vi "MVMT.vi"() -> ()   [LabVIEW 2011]
uses:
  <vilib>/vision/Pattern Matching.llb/IMAQ Curve Parameters.ctl
  <vilib>/vision/Analysis.llb/IMAQ ExtractCurvesCurve.ctl
  <vilib>/Platform/TimedLoop/XDataNode/timing_clust.ctl
  <vilib>/Platform/TimedLoop/XDataNode/nitl_modes.ctl
  <vilib>/Platform/TimedLoop/XDataNode/wakeup.ctl
  <vilib>/Platform/TimedLoop/XDataNode/XDataNode.xnode
  <vilib>/vision/NI_Vision_Development_Module.lvlib
  <vilib>/Platform/TimedLoop/XDataNode/XDNodeRunTimeDep.lvlib
panel:
  in  "Median Filter Size":i32=5 min=0 max=7
  in  "Distance to Camera Visible":cluster{dbl, dbl}(slide)={0.0, 3.88} scale=0.0..3.0
  out "Curves":T1[](array[typedef]) {"Points"."Y" format="%.2f"; "Points"."X" format="%.2f"}
  out "Image":T2(plugin-control)
  in  "Curve Parameters":T3={"Extraction Mode"=1, "Edge Threshold"=1, "Edge Filter Size"=0, "Min Length"=25, "Row Search Step Size"=15, "Col Search Step Size"=15, "Max Endpoint Gap"=10, "Closed"=TRUE, "Subpixel"=TRUE} {"Extraction Mode" items=["Normal", "Uniform Regions"]; "Edge Filter Size" items=["Fine", "Normal", "Contour Tracing"]; "Max Endpoint Gap" min=0; "Col Search Step Size" min=1 max=255 step=1; "Row Search Step Size" min=1 max=255 step=1; "Min Length" min=0; "Edge Threshold" min=1 max=350 step=1}
  in  "Range":cluster{"Lower value":sgl, "Upper value":sgl}={"Lower value"=0.05, "Upper value"=10.0} {"Upper value" format="%.2f"; "Lower value" format="%.2f"}
  in  "Zero Out Baseline":bool
  in  "Status":string
  in  "Start":bool
  out "Frame Display":T2(plugin-control)
  in  "# Frames in Average":i32=100
  in  "stop":bool
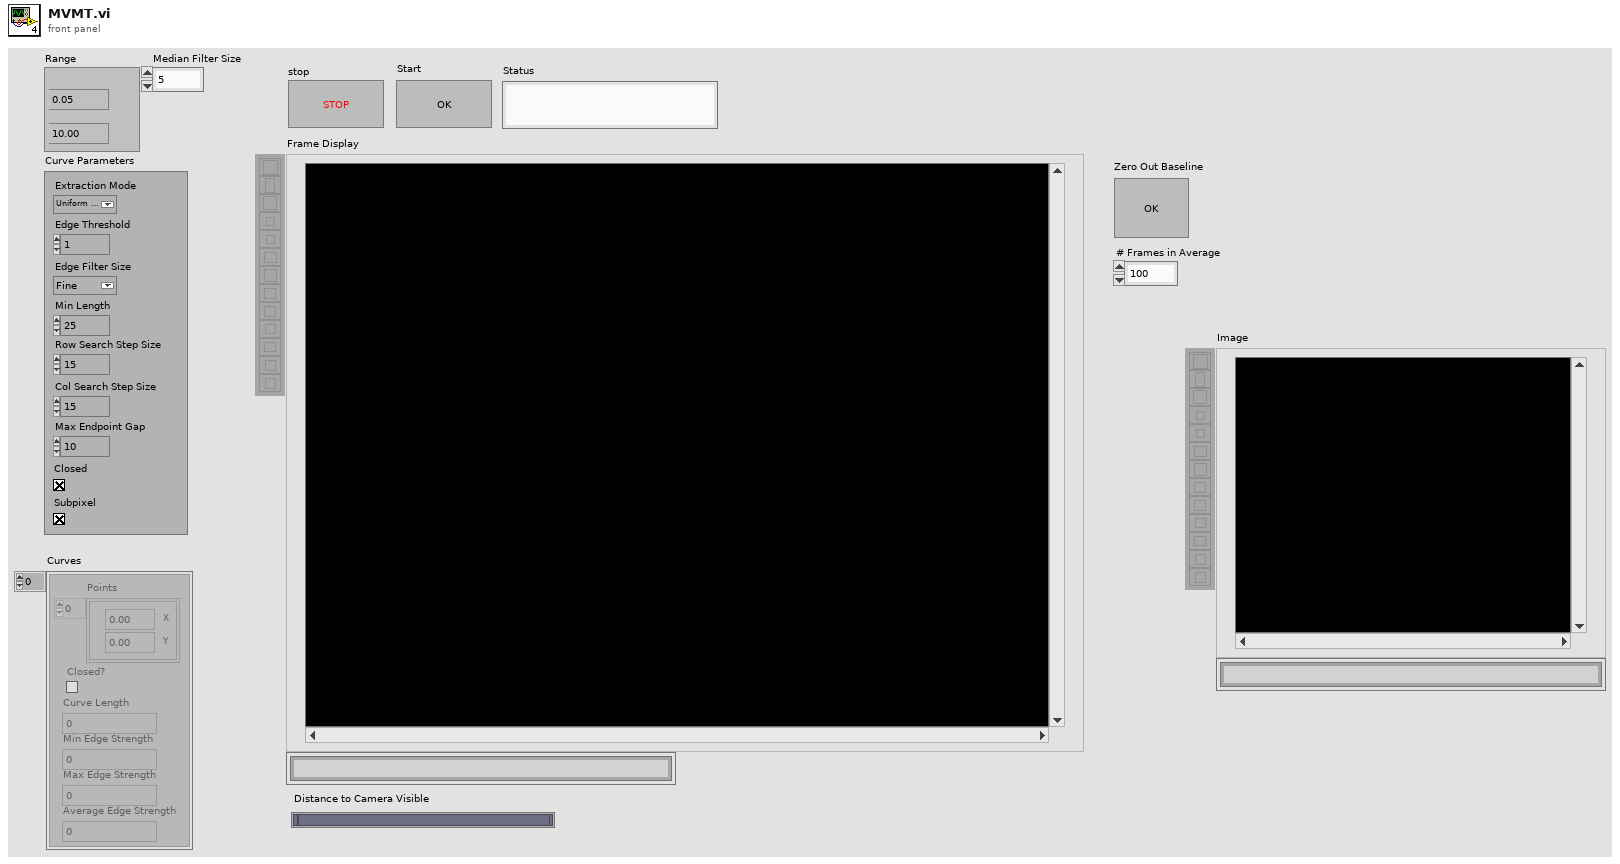
[diagram p1: front panel]
types:
  T1 = typedef "IMAQ ExtractCurvesCurve.ctl" = cluster{"Points":cluster{"X":dbl, "Y":dbl}[], "Closed?":bool, "Curve Length":dbl, "Min Edge Strength":dbl, "Max Edge Strength":dbl, "Average Edge Strength":dbl}
  T2 = typedef "IMAQ Image.ctl" = refnum<image>
  T3 = typedef "IMAQ Curve Parameters.ctl" = cluster{"Extraction Mode":u32, "Edge Threshold":i32, "Edge Filter Size":u32, "Min Length":i32, "Row Search Step Size":i32, "Col Search Step Size":i32, "Max Endpoint Gap":i32, "Closed":bool, "Subpixel":bool}
  T4 = enum16{"Record", "Idle", "Acquire Background", "Stop"}
  T5 = typedef "t_CallbackReferences.ctl" = cluster{"LV event callback ":refnum<k27>, "Proxy instance":refnum<k24>, "(*f)(...)":i32}
  T6 = typedef "XDNodeRunTimeDep.lvlib/timing_clust.ctl" = cluster{"Expected End [f-1]":u64, "Actual End [f-1]":u64, "Finished Late? [f-1]":bool, "Expected End [i-1]":u64, "Actual End [i-1]":u64, "Finished Late? [i-1]":bool, "Expected Start [i]":u64, "Actual Start [i]":u64, "Expected Start [f]":u64, "Actual Start [f]":u64, "Source Name":string, "Structure Name":string, "Period":i64, "Deadline":i64, "Offset":i64, "Start":i64, "Priority":i32, "Timeout":i32, "Mode":T7, "Wakeup Reason":T8, "Error":errorcluster, "Source Type":string, "Secondary Source Type":string, "Global End Time":u64, "Global Start Time":u64, "Frame Duration":u64, "Iteration Duration":u64, "Assigned CPU":i32, "I/O Scan Engine Mode":u32}
  T7 = typedef "XDNodeRunTimeDep.lvlib/nitl_modes.ctl" = enum32{"No Change", "Process missed periods, maintain original phase", "Discard missed periods, maintain original phase", "Process missed periods, ignore original phase", "Discard missed periods, ignore original phase"}
  T8 = typedef "XDNodeRunTimeDep.lvlib/wakeup.ctl" = enum32{"Normal", "Aborted", "Asynchronous wakeup", "Timing source error", "Timed loop error", "Timeout"}
  T9 = enum32{"Average", "Min", "Max", "Clear  if < ", "Clear  if < or =", "Clear  if =", "Clear  if > or =", "Clear  if >"}
  T10 = typedef "Image Type" = u32
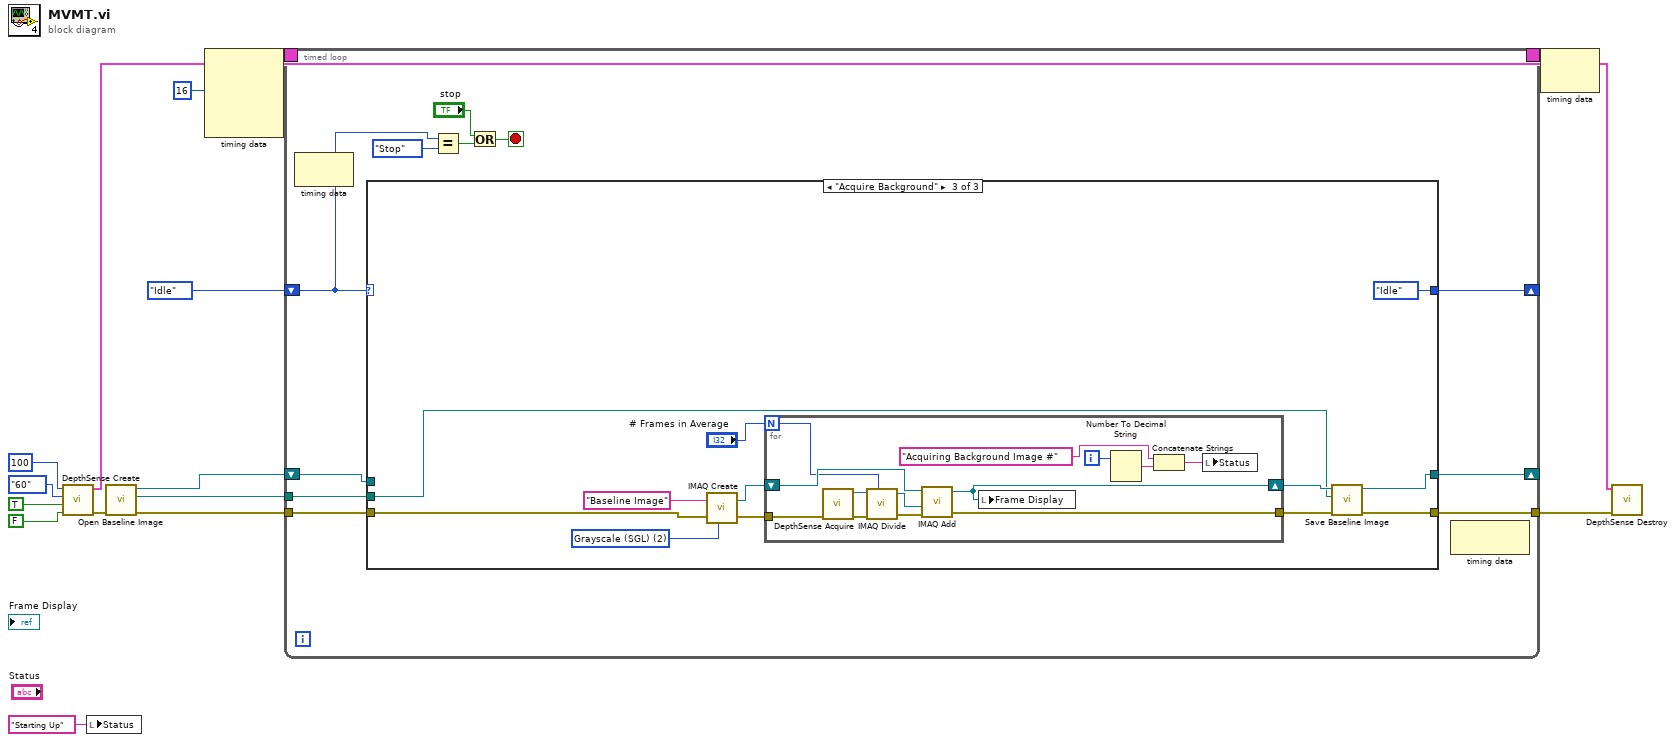
[diagram p0: block diagram]
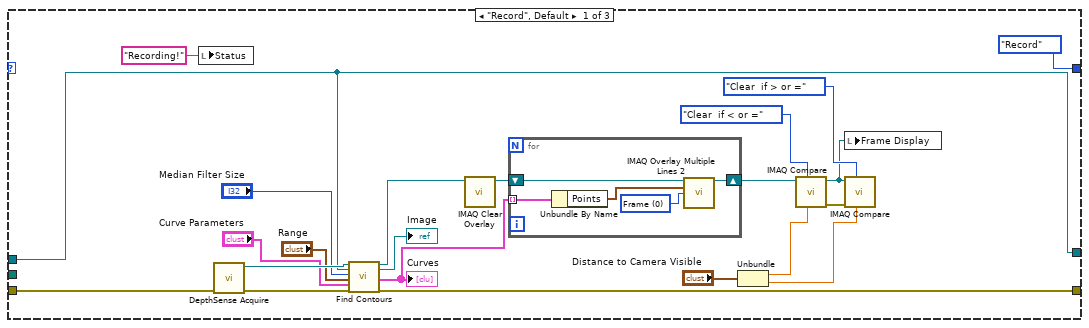
[diagram p2: hidden frame]
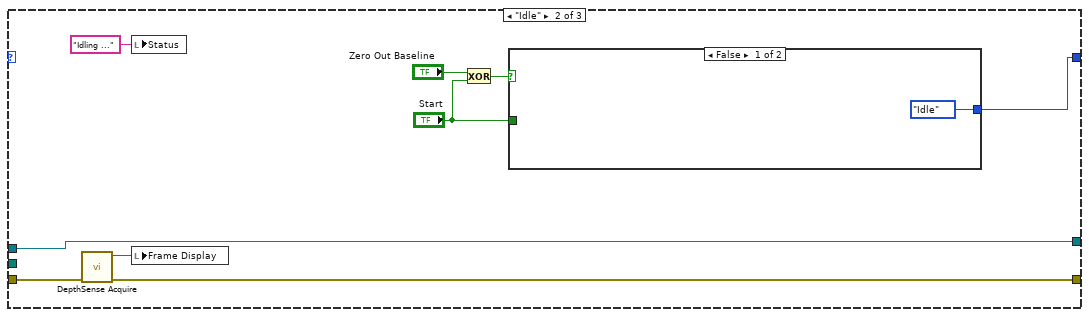
[diagram p3: hidden frame]
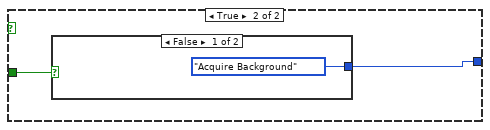
[diagram p4: hidden frame]
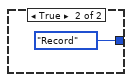
[diagram p5: hidden frame]
diagram:
  n1 = call "DepthSense Create.vi"("Denoise?"=FALSE, "Close Mode?"=TRUE, "Framerate"=enum32{"25", "30", "50", "60"}."60", "Confidence"=100) -> ("error out"=w5:errorcluster, "callbacks"=w1:cluster{"References":T5, "References":T5})  [unwired: 5 in, 1 out]
  n2 = local write "Status"("Starting Up" ("Status")) -> ()
  n3 = call "Open Baseline Image.vi"("error in (no error)"=w5) -> ("error out"=w4:errorcluster, "dup path"=w3:path, "Image Out"=w2:T2)  [unwired: 8 in]
  n4 = node-c288(i64 16 ("Period")) -> (w9:T6)  [unwired: 3 in]
  n5 = timed-loop {
    tunnel: w4 -> [w26]
    tunnel: [w25] -> w15
    shift-right: [w18] -> _
    shift-left: T4."Idle" -> [w20]
    shift-right: [w17] -> _
    shift-left: w2 -> [w24]
    tunnel: w3 -> [w16]
    timing: w9 -> [_]
    timing-out: [_] -> w8
    stop <- w22 stop-if-true
    n6 = node-c288() -> ()  [unwired: 1 in, 1 out]
    n7 = case shown="\"Acquire Background\"" w20 {
      tunnel: w26 -> [w50 w64 w77]
      tunnel: [w48 w63 w73] -> w25
      tunnel: w24 -> [w43 w61 _]
      tunnel: [T4."Record" w57 T4."Idle"] -> w18
      tunnel: [w43 w61 w70] -> w17
      tunnel: w16 -> [_ _ w71]
      frame "Record", Default {
        n8 = local write "Status"("Recording!" ("Status")) -> ()
        n9 = call "DepthSense Acquire.vi"("error in (no error)"=w50) -> ("error out"=w44:errorcluster, "new depth frame"=w47:T2)  [unwired: 9 in]
        n10 = call "Find Contours.vi"("Image Src"=w47, "Background Image"=w43, "Median Filter Size"="Median Filter Size", "Range"="Range", "Curve Parameters"="Curve Parameters", "error in (no error)"=w44) -> ("Image Src Dup"=w42:T2, "Background Subtracted Image"=→"Image":T2, "Curves"=w39:T1[], "error out"=w48:errorcluster)  [unwired: 10 in]
        "Curves" <- w39
        n11 = call "IMAQ Clear Overlay"("Image"=w42) -> ("Image Out"=w41:T2)  [unwired: 9 in, 1 out]
        n12 = for {
          tunnel: w39 -> [w55] mode=indexing
          shift-right: [w51] -> w38
          shift-left: w41 -> [w54]
          w52 = u32 0 items=["Frame", "Fill"] ("Drawing Mode (Frame)")
          n13 = Unbundle By Name(w55) -> ("Points"=w53:cluster{"X":dbl, "Y":dbl}[])
          n14 = call "IMAQ Overlay Multiple Lines 2"("Image"=w54, "Line End Points"=w53, "Drawing Mode (Frame)"=w52) -> ("Image Out"=w51:T2)  [unwired: 11 in, 1 out]
        }
        n15 = Unbundle("Distance to Camera Visible") -> (w32:dbl, w31:dbl)
        n16 = call "IMAQ Compare"("Constant"=w32, "Operator"=T9."Clear  if < or =", "Image Src A"=w38) -> ("error out"=w35:errorcluster, "Image Dst Out"=w34:T2)  [unwired: 7 in]
        n17 = local write "Frame Display"(w34) -> ()
        n18 = call "IMAQ Compare"("Constant"=w31, "Operator"=T9."Clear  if > or =", "error in (no error)"=w35, "Image Src A"=w34) -> ()  [unwired: 6 in, 2 out]
      }
      frame "Idle" {
        n19 = call "DepthSense Acquire.vi"("error in (no error)"=w64) -> ("error out"=w63:errorcluster, "new depth frame"=w56:T2)  [unwired: 9 in]
        n20 = local write "Status"("Idling ..." ("Status")) -> ()
        n21 = local write "Frame Display"(w56) -> ()
        n22 = Exclusive Or(1:"Start", 2:"Zero Out Baseline") -> (0:w59:bool)
        n23 = case shown="False" w59 {
          tunnel: "Start" -> [_ w67]
          tunnel: [T4."Idle" w66] -> w57
          frame False {
          }
          frame True {
            n24 = case shown="False" w67 {
              tunnel: [T4."Acquire Background" T4."Record"] -> w66
              frame False {
              }
              frame True {
              }
            }
          }
        }
      }
      frame "Acquire Background" {
        w80 = T10 2 items=["Grayscale (U8)", "Grayscale (I16)", "Grayscale (SGL)", "Complex (CSG)", "RGB (U32)", "HSL (U32)", "RGB (U64)", "Grayscale (U16)"] ("Image Type")
        n25 = call "IMAQ Create"("Image Name"="Baseline Image", "Image Type"=w80, "error in (no error)"=w77) -> ("New Image"=w79:T2, "error out"=w76:errorcluster)  [unwired: 2 in]
        n26 = for {
          N: "# Frames in Average" -> [w83]
          tunnel: w76 -> [w94]
          shift-right: [w82] -> w72
          shift-left: w79 -> [w91]
          tunnel: [w89] -> w74
          i -> [w85]
          n27 = call "DepthSense Acquire.vi"("error in (no error)"=w94) -> ("error out"=w93:errorcluster, "new depth frame"=w92:T2)  [unwired: 9 in]
          n28 = call "IMAQ Divide"("Image Src A"=w92, "Constant"=w83, "error in (no error)"=w93) -> ("Image Dst Out"=w84:T2, "error out"=w90:errorcluster)  [unwired: 4 in]
          n29 = call "IMAQ Add"("Image Src A"=w91, "Image Src B"=w84, "error in (no error)"=w90) -> ("Image Dst Out"=w82:T2, "error out"=w89:errorcluster)  [unwired: 4 in]
          n30 = local write "Frame Display"(w82) -> ()
          n31 = Number To Decimal String(number=w85) -> (decimal integer string=w88:string)  [unwired: 1 in]
          n32 = Concatenate Strings("Acquiring Background Image #" ("Status"), w88) -> (w86:string)
          n33 = local write "Status"(w86) -> ()
        }
        n34 = call "Save Baseline Image.vi"("error in (no error)"=w74, "Baseline Image Path"=w71, "Baseline Image"=w72) -> ("error out"=w73:errorcluster, "Baseline Image Out"=w70:T2)  [unwired: 7 in]
      }
    }
    n35 = Equal?(x=w20, y=T4."Stop") -> (x = y?=w21:bool)
    n36 = Or(x="stop", y=w21) -> (x .or. y?=w22:bool)
    n37 = node-c288() -> ()  [unwired: 1 in, 1 out]
  }
  n38 = node-c288(w8) -> ()  [unwired: 1 out]
  n39 = call "DepthSense Destroy.vi"("error in (no error)"=w15, "callbacks"=w1) -> ()  [unwired: 10 in]
